vi "Threshold with Hysteresis 2.vi"(6 "Threshold Lo":dbl=-250.0, 7 "Threshold Hi":dbl, 8 "Input Dif":dbl(slide)=313.0 step=1.0 scale=-1000.0..1000.0 scale format="%1.1f") -> (2 "Power  Out":bool, 3 "Out Dif Last":dbl=313.0)   [LabVIEW 2011]
doc: "Use this template to build a standard state machine design pattern. Each state executes code and determines which state to transition to. Contrast this design pattern with the User Interface Event Handler pattern, in which code executes in response to user actions. Contrast this design pattern also with the Queued Message Handler pattern, in which each message handling code can queue zero or more new messages."
panel:
  in  "Power  In":bool
  out "Between":bool
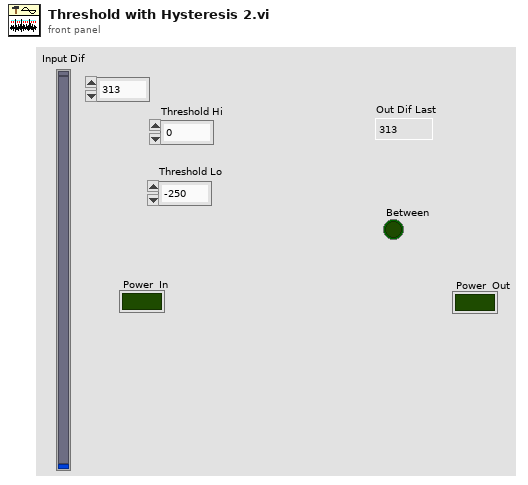
[diagram p1: front panel]
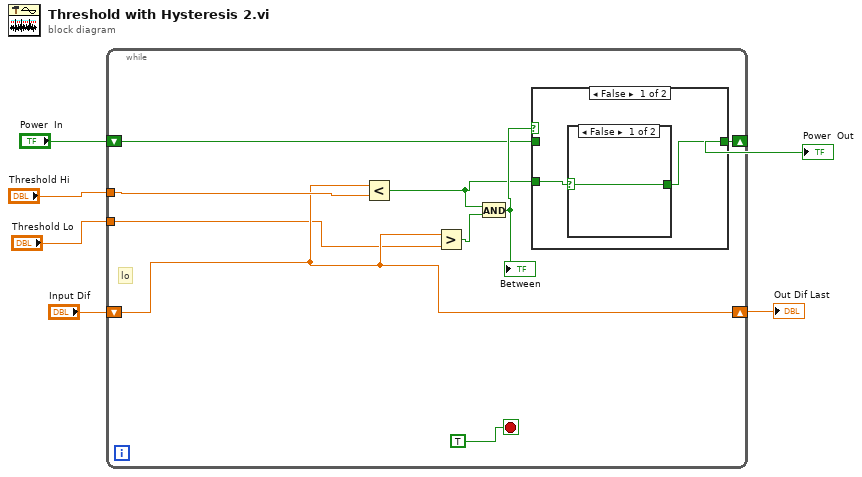
[diagram p0: block diagram]
diagram:
  n1 = while {
    tunnel: "Threshold Hi" -> [w14]
    tunnel: "Threshold Lo" -> [w12]
    shift-right: [w13] -> w3
    shift-left: "Input Dif" -> [w13]
    shift-right: [w8] -> w1
    shift-left: "Power  In" -> [w9]
    stop <- TRUE ("Boolean") stop-if-true
    # "lo"
    n2 = Less?(x=w13, y=w14) -> (x < y?=w7:bool)
    n3 = Greater?(x=w13, y=w12) -> (0:w11:bool)
    n4 = And(x=w7, y=w11) -> (x .and. y?=w10:bool)
    "Between" <- w10
    n5 = case shown="False" w10 {
      tunnel: w9 -> [_ w20]
      tunnel: [w16 w20] -> w8
      tunnel: w7 -> [w17 _]
      frame False {
        n6 = case shown="False" w17 {
          selector: w17 -> [w18 w19]
          tunnel: [w18 w19] -> w16
          frame False {
          }
          frame True {
          }
        }
      }
      frame True {
      }
    }
  }
  "Out Dif Last" <- w3
  "Power  Out" <- w1
